vi "Aim subvi.vi"(0 "Coordinates":cluster{"X":i32, "Y":i32}, 3 "error in (no error)":errorcluster) -> (6 "Cluster 3":cluster{"X":i32, "Y":i32}, 7 "Cluster 2":cluster{"X":i32, "Y":i32}, 8 "Cluster 4":cluster{"X":i32, "Y":i32}, 9 "Cluster":cluster{"X":i32, "Y":i32}, 10 "error out":errorcluster)   [LabVIEW 2020]
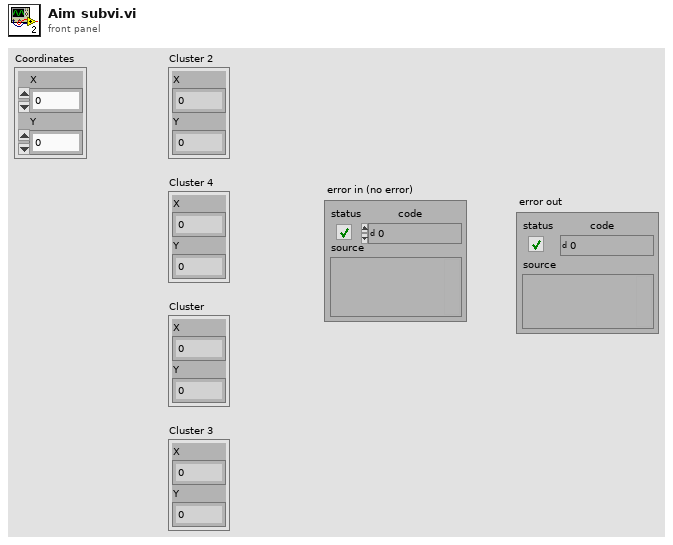
[diagram p1: front panel]
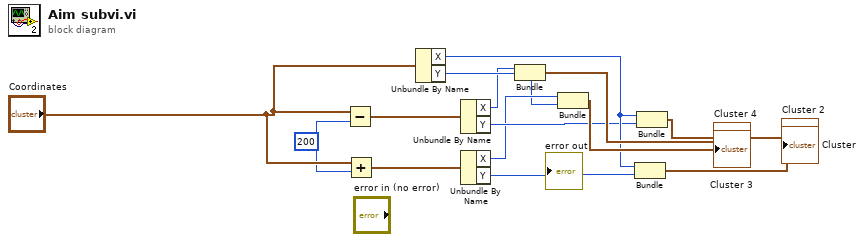
[diagram p0: block diagram]
diagram:
  w9 = 200
  n1 = Subtract(x="Coordinates", y=w9) -> (x-y=w1:cluster{"X":i32, "Y":i32})
  n2 = Add(x="Coordinates", y=w9) -> (x+y=w2:cluster{"X":i32, "Y":i32})
  n3 = Unbundle By Name("Coordinates") -> ("X"=w8:i32, "Y"=w4:i32)
  n4 = Unbundle By Name(w1) -> ("X"=w3:i32, "Y"=w7:i32)
  n5 = Unbundle By Name(w2) -> ("X"=w5:i32, "Y"=w6:i32)
  n6 = Bundle("X"=w3, "Y"=w4) -> (→"Cluster 4":cluster{"X":i32, "Y":i32})  [unwired: 1 in]
  n7 = Bundle("X"=w5, "Y"=w4) -> (→"Cluster 3":cluster{"X":i32, "Y":i32})  [unwired: 1 in]
  n8 = Bundle("X"=w8, "Y"=w6) -> (→"Cluster":cluster{"X":i32, "Y":i32})  [unwired: 1 in]
  n9 = Bundle("X"=w8, "Y"=w7) -> (→"Cluster 2":cluster{"X":i32, "Y":i32})  [unwired: 1 in]
